vi "svc_Caller VI Returned in Error Source.vi"(3 "warning input to caller":errorcluster, 4 "error in (no error)":errorcluster) -> (1 "error out":errorcluster)   [LabVIEW 2017]
panel:
  # "This VI must be called as a subVI to be useful.  It should be dropped\nin whatever VI should be the \"origin\" of the error."
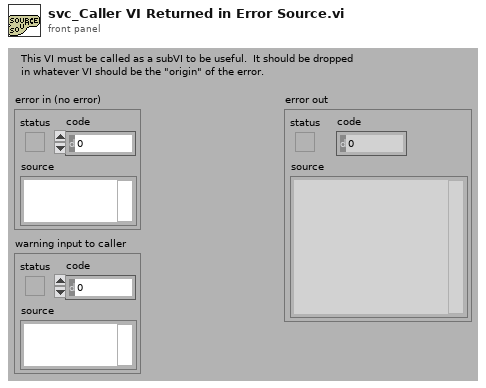
[diagram p1: front panel]
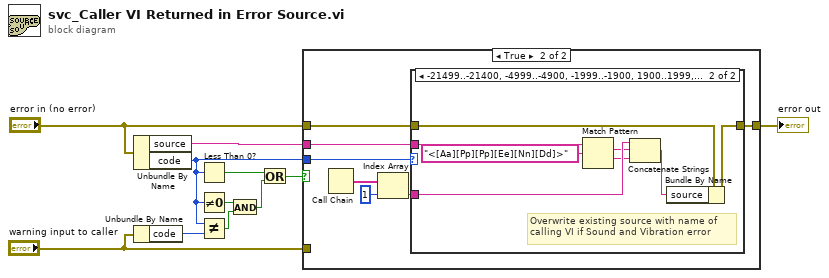
[diagram p0: block diagram]
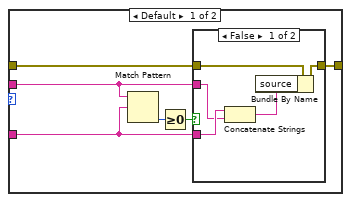
[diagram p3: hidden frame]
diagram:
  n1 = Unbundle By Name("error in (no error)") -> ("source"=w1:string, "code"=w2:i32)
  n2 = Unbundle By Name("warning input to caller") -> ("code"=w8:i32)
  n3 = Less Than 0?(x=w2) -> (x < 0?=w7:bool)
  n4 = Not Equal To 0?(x=w2) -> (x != 0?=w5:bool)
  n5 = Not Equal?(x=w2, y=w8) -> (x != y?=w4:bool)
  n6 = And(x=w5, y=w4) -> (x .and. y?=w3:bool)
  n7 = Or(x=w7, y=w3) -> (x .or. y?=w6:bool)
  n8 = case shown="True" w6 {
    tunnel: "error in (no error)" -> [_ w19]
    tunnel: [w12 w16] -> w10
    tunnel: "warning input to caller" -> [w12 _]
    tunnel: w2 -> [_ w18]
    tunnel: w1 -> [_ w17]
    frame False {
    }
    frame True {
      n9 = Call Chain() -> (call chain=w15:string[])
      n10 = Index Array(array=w15, index=1 ("Index")) -> (element=w13:string)
      n11 = case shown="-21499..-21400, -4999..-4900, -1999..-1900, 1900..1999, 4900..4999, 21400..21499" w18 {
        tunnel: w19 -> [w21 w39]
        tunnel: [w20 w38] -> w16
        tunnel: w17 -> [w23 w37]
        tunnel: w13 -> [w22 w35]
        frame Default {
          n12 = Match Pattern(string=w23, regular expression=w22) -> (offset past match=w25:i32)  [unwired: 1 in, 3 out]
          n13 = Greater Or Equal To 0?(x=w25) -> (x >= 0?=w24:bool)
          n14 = case shown="False" w24 {
            tunnel: w23 -> [w29 _]
            tunnel: w22 -> [w30 _]
            tunnel: w21 -> [w28 w31]
            tunnel: [w27 w31] -> w20
            frame False {
              n15 = Concatenate Strings(w30, w29) -> (w26:string)
              n16 = Bundle By Name(cluster=w28, "source"=w26) -> (w27:errorcluster)
            }
            frame True {
            }
          }
        }
        frame -21499..-21400, -4999..-4900, -1999..-1900, 1900..1999, 4900..4999, 21400..21499 {
          # "Overwrite existing source with name of\ncalling VI if Sound and Vibration error"
          n17 = Match Pattern(string=w37, regular expression="<[Aa][Pp][Pp][Ee][Nn][Dd]>") -> (match substring=w34:string, after substring=w33:string)  [unwired: 1 in, 2 out]
          n18 = Concatenate Strings(w35, w34, w33) -> (w32:string)
          n19 = Bundle By Name(cluster=w39, "source"=w32) -> (w38:errorcluster)
        }
      }
    }
  }
  "error out" <- w10
